vi "Determine Nim data type.vi"(8 "error in (no error)":errorcluster, 11 "String":string) -> (0 "error out":errorcluster, 3 "Nim data type":T1)   [LabVIEW 2013]
uses:
  Nim data types.ctl
panel:
  in  "Nim data types":T1=enum."meid"
  out "Is BTW Serial Number?":bool
  out "Is BTWSSWWYY?":bool
  out "Is MAC without semicolons":bool
  out "Is MAC with semicolons?":bool
  out "Is MEID?":bool
  out "Is CCID?":bool
  out "Is IMEI?":bool
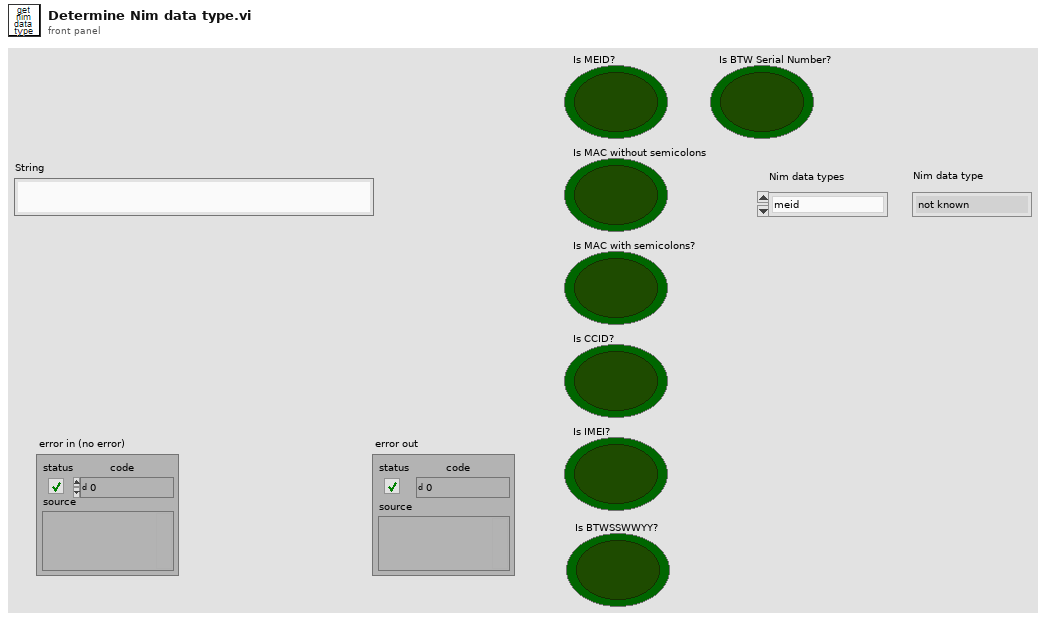
[diagram p1: front panel]
types:
  T1 = typedef "Nim data types.ctl" = enum16{"not known", "meid", "mac with semis", "mac no semis", "ccid", "imei", "btwsswwyy", "btw serial number"}
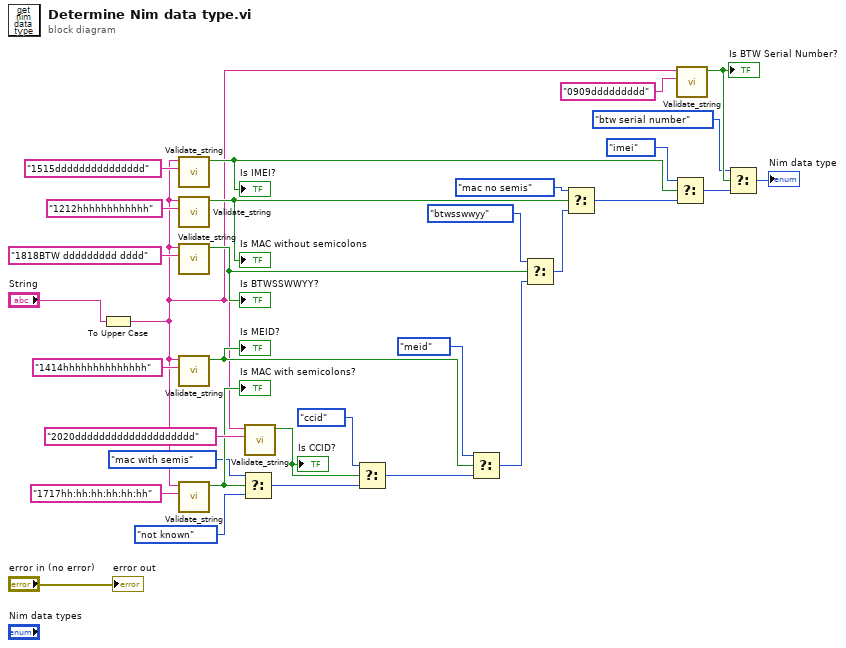
[diagram p0: block diagram]
diagram:
  n1 = To Upper Case(1:"String") -> (0:w1:string)
  n2 = call "Validate_string.vi"("String data format"="1515ddddddddddddddd", "String"=w1) -> ("String Valid"=w20:bool)  [unwired: 8 in, 1 out]
  "Is IMEI?" <- w20
  n3 = call "Validate_string.vi"("String data format"="1212hhhhhhhhhhhh", "String"=w1) -> ("String Valid"=w19:bool)  [unwired: 8 in, 1 out]
  "Is MAC without semicolons" <- w19
  n4 = call "Validate_string.vi"("String data format"="1818BTW ddddddddd dddd", "String"=w1) -> ("String Valid"=w18:bool)  [unwired: 8 in, 1 out]
  "Is BTWSSWWYY?" <- w18
  n5 = call "Validate_string.vi"("String data format"="1414hhhhhhhhhhhhhh", "String"=w1) -> ("String Valid"=w17:bool)  [unwired: 8 in, 1 out]
  "Is MEID?" <- w17
  n6 = call "Validate_string.vi"("String data format"="1717hh:hh:hh:hh:hh:hh", "String"=w1) -> ("String Valid"=w24:bool)  [unwired: 8 in, 1 out]
  "Is MAC with semicolons?" <- w24
  n7 = Select(t=Nim_data_types."mac with semis" ("Nim data type"), s=w24, f=Nim_data_types."not known" ("Nim data type")) -> (s? t:f=w5:T1)
  n8 = call "Validate_string.vi"("String data format"="2020dddddddddddddddddddd", "String"=w1) -> ("String Valid"=w16:bool)  [unwired: 8 in, 1 out]
  "Is CCID?" <- w16
  n9 = Select(t=Nim_data_types."ccid" ("Nim data type"), s=w16, f=w5) -> (s? t:f=w6:T1)
  n10 = Select(t=Nim_data_types."meid" ("Nim data type"), s=w17, f=w6) -> (s? t:f=w7:T1)
  n11 = Select(t=Nim_data_types."btwsswwyy" ("Nim data type"), s=w18, f=w7) -> (s? t:f=w8:T1)
  n12 = Select(t=Nim_data_types."mac no semis" ("Nim data type"), s=w19, f=w8) -> (s? t:f=w9:T1)
  n13 = Select(t=Nim_data_types."imei" ("Nim data type"), s=w20, f=w9) -> (s? t:f=w10:T1)
  n14 = call "Validate_string.vi"("String data format"="0909ddddddddd", "String"=w1) -> ("String Valid"=w22:bool)  [unwired: 8 in, 1 out]
  "Is BTW Serial Number?" <- w22
  n15 = Select(t=Nim_data_types."btw serial number" ("Nim data type"), s=w22, f=w10) -> (s? t:f=→"Nim data type":T1)
  "error out" <- "error in (no error)"
